vi "Actor Core.vi"(8 "error in":errorcluster, 11 "UDP_receiver in":refnum<class "UDP_receiver.lvclass">) -> (0 "error out":errorcluster, 3 "Actor out":refnum<class "Actor.lvclass">)   [LabVIEW 2025, in "UDP_receiver.lvlib" / "UDP_receiver.lvclass"]
doc: "(<B>Filename</B>: Actor Framework.lvlib:Actor.lvclass:Actor Core.vi)\n\nReceives messages to the actor, reacts to them, and initiates any error handling that may shut the actor down.\n\nDescendant classes may override this VI to append parallel tasks for the actor to complete while it handles messages. Overrides use the Call Parent Class Method node."
uses:
  UDP_receiver.lvclass
  C:/Program Files/National Instruments/LabVIEW 2025/vi.lib/ActorFramework/Actor/Actor.lvclass
  <vilib>/ActorFramework/Actor/Actor.lvclass
  UDP_receiver.lvclass/UDP_receiver.ctl
  <vilib>/ActorFramework/Actor/Actor.lvclass/Actor.ctl
  <vilib>/ActorFramework/Message Enqueuer/Message Enqueuer.lvclass/Message Enqueuer.ctl
  UDP_receiver Messages/data_to_parser Msg/data_to_parser Msg.lvclass/data_to_parser Msg.ctl
  <vilib>/ActorFramework/Message Enqueuer/Init from Existing Queue.vi
  <vilib>/ActorFramework/Message Enqueuer/Enqueue.vi
  <vilib>/ActorFramework/Stop Msg/Stop Msg.lvclass
  C:/Program Files/National Instruments/LabVIEW 2025/vi.lib/ActorFramework/Message/Message.lvclass
  UDP_receiver Messages/data_to_parser Msg/data_to_parser Msg.lvclass
  <vilib>/ActorFramework/Message Priority Queue/Priority Enqueue.vi
  <vilib>/ActorFramework/Message Enqueuer/Message Enqueuer.lvclass
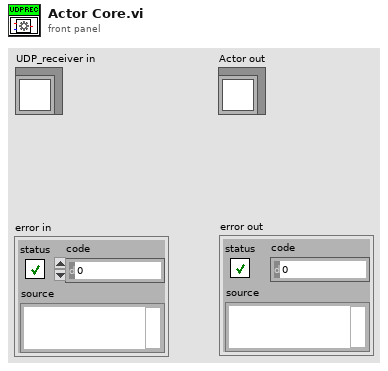
[diagram p1: front panel]
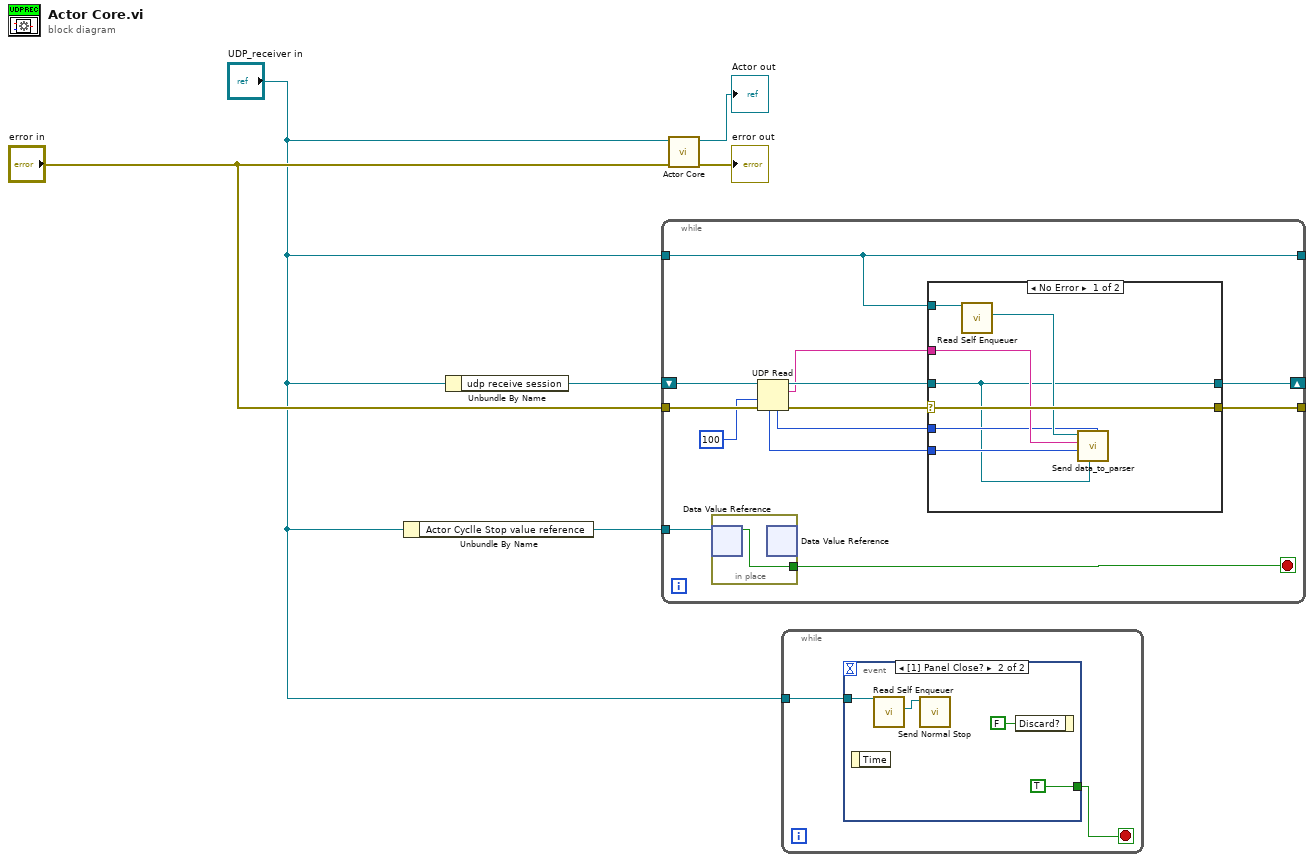
[diagram p0: block diagram]
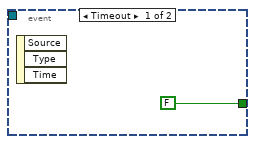
[diagram p2: hidden frame]
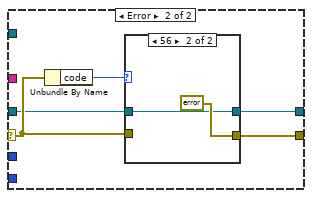
[diagram p3: hidden frame]
diagram:
  n1 = Unbundle By Name("UDP_receiver in") -> ("Actor Cyclle Stop value reference"=w2:refnum<data-value>)
  n2 = Unbundle By Name("UDP_receiver in") -> ("udp receive session"=w3:refnum<k16>)
  n3 = while {
    tunnel: "UDP_receiver in" -> [w7]
    tunnel: "error in" -> [w18]
    shift-right: [w14] -> _
    shift-left: w3 -> [w19]
    tunnel: [w12] -> _
    tunnel: [w7] -> _
    tunnel: w2 -> [w11]
    stop <- w10 stop-if-true
    n4 = in-place {
      in-place-border: [w20] -> w10
      n5 = in-place-dvr #1(w11) -> (w20:bool)  [unwired: 1 out]
      n6 = in-place-dvr #1() -> ()  [unwired: 1 in, 2 out]
    }
    n7 = UDP Read(connection ID=w19, timeout ms (25000)=100, 8:w18) -> (data out=w13:string, error out=w16:errorcluster, 3:w15:refnum<k16>, 4:w9:u16, 6:w8:u32)  [unwired: 1 in]
    n8 = case shown="No Error" w16 {
      selector: w16 -> [w27 w31]
      tunnel: w15 -> [w21 w29]
      tunnel: [w21 w28] -> w14
      tunnel: w13 -> [w24 _]
      tunnel: [w27 w30] -> w12
      tunnel: w9 -> [w22 _]
      tunnel: w8 -> [w23 _]
      tunnel: w7 -> [w26 _]
      frame No Error {
        n9 = call <vilib>:"Read Self Enqueuer.vi"("Actor"=w26) -> ("Self Enqueuer"=w25:refnum<class "Message Enqueuer.lvclass">)  [unwired: 10 in]
        n10 = call "Send data_to_parser.vi"("port"=w22, "connection ID out"=w21, "address"=w23, "udp message"=w24, "Message Enqueuer"=w25) -> ()  [unwired: 5 in, 2 out]
      }
      frame Error {
        n11 = Unbundle By Name(w31) -> ("code"=w32:i32)
        n12 = case shown="56" w32 {
          tunnel: w31 -> [w34 _]
          tunnel: [w34 errorcluster {"status"=FALSE, "code"=0, "source"=""} ("error IO")] -> w30
          tunnel: w29 -> [w33 w35]
          tunnel: [w33 w35] -> w28
          frame 0, Default {
          }
          frame 56 {
          }
        }
      }
    }
  }
  n13 = call-parent "Actor Core.vi"("error in"="error in", "Actor in"="UDP_receiver in") -> ("error out"=→"error out":errorcluster, "Actor out"=→"Actor out":refnum<class "Actor.lvclass">)  [unwired: 8 in]
  n14 = while {
    tunnel: "UDP_receiver in" -> [w38]
    stop <- w37 stop-if-true
    n15 = event shown="[1] Panel Close?" {
      selector: _ -> [_ _]
      dyn-events: _ -> [_ _]
      timeout: _ -> [_ _]
      tunnel: w38 -> [_ w43]
      tunnel: [FALSE TRUE] -> w37
      event Timeout {
        n16 = event-data() -> ()  [unwired: 1 in, 3 out]
      }
      event Panel Close? {
        n17 = event-data() -> ()  [unwired: 1 in, 1 out]
        n18 = call <vilib>:"Read Self Enqueuer.vi"("Actor"=w43) -> ("Self Enqueuer"=w42:refnum<class "Message Enqueuer.lvclass">)  [unwired: 10 in]
        n19 = call <vilib>:"Send Normal Stop.vi"("Message Enqueuer"=w42) -> ()  [unwired: 10 in, 1 out]
        n20 = event-data("Discard?"=FALSE) -> ()  [unwired: 1 in, 1 out]
      }
    }
  }
